vi "004 Local variable exemple.vi"() -> ()   [LabVIEW 2019]
panel:
  in  "OK Button":bool
  out "Value":dbl
  out "Local Var":dbl
  in  "Color":u32(colorbox)
  in  "Disabled":T1(ring)
  in  "Visible":bool
  in  "Numeric":dbl
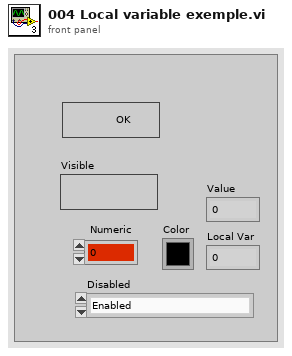
[diagram p1: front panel]
types:
  T1 = enum8{"Enabled", "Disabled", "Disabled and Grayed Out"}
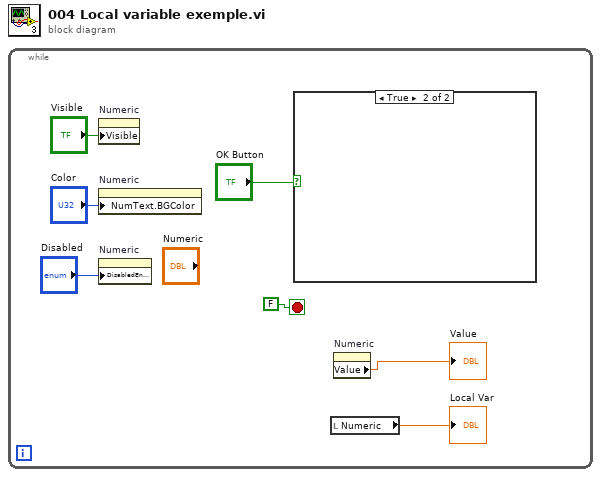
[diagram p0: block diagram]
diagram:
  n1 = while {
    stop <- FALSE stop-if-true
    n2 = property on="Numeric" class="DigNum (strict)"("Visible"="Visible") -> ()  [unwired: 2 in, 2 out]
    n3 = property on="Numeric" class="DigNum (strict)"("NumText.BGColor"="Color") -> ()  [unwired: 2 in, 2 out]
    n4 = property on="Numeric" class="DigNum (strict)"("DisabledEnum"="Disabled") -> ()  [unwired: 2 in, 2 out]
    n5 = case shown="True" "OK Button" {
      frame False {
      }
      frame True {
      }
    }
    n6 = local read "Numeric"() -> (→"Local Var":dbl)
    n7 = property on="Numeric" class="DigNum (strict)"() -> ("Value"=→"Value":dbl)  [unwired: 2 in, 2 out]
  }
